vi "testPythonResults.vi"() -> ()   [LabVIEW 2011, in "run.lvlib"]
uses:
  run.lvlib
  Tools/Filing/FileReader/FileReader.lvclass
  Channels/Digital/DigitalOutput.lvclass
  Channels/DDSOutput/Generic/DDSOutput.lvclass
  Channels/VoltOutput/AnalogOutput.lvclass
panel:
  out "times":dbl[](array[numeric]) format="%#_6f"
  in  "Device":T1(ring)
  out "data":dbl[][](array[numeric])
  in  "Path":path=path "C:/Users/Administrator/Desktop/Crete/Data/2014/1411/141126/Scripts/Instrument Scripts/Dio64.csv"
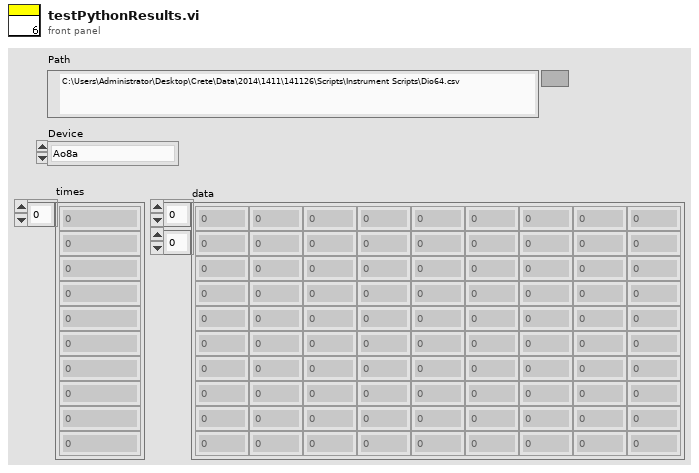
[diagram p1: front panel]
types:
  T1 = enum16{"Ao8a", "Ao8b", "Dio64", "K2602a", "K2602b", "K2602c", "K2602d", "SpinCoreDDS0", "SpinCoreDDS1"}
  T2 = cluster{"aoChannels":refnum<class "AnalogOutput.lvclass">[], "doChannels":refnum<class "DigitalOutput.lvclass">[], "rfChannels":refnum<class "DDSOutput.lvclass">[]}
  T3 = cluster{"Timestamps ms":dbl[], "DataPerChannel":dbl[][]}
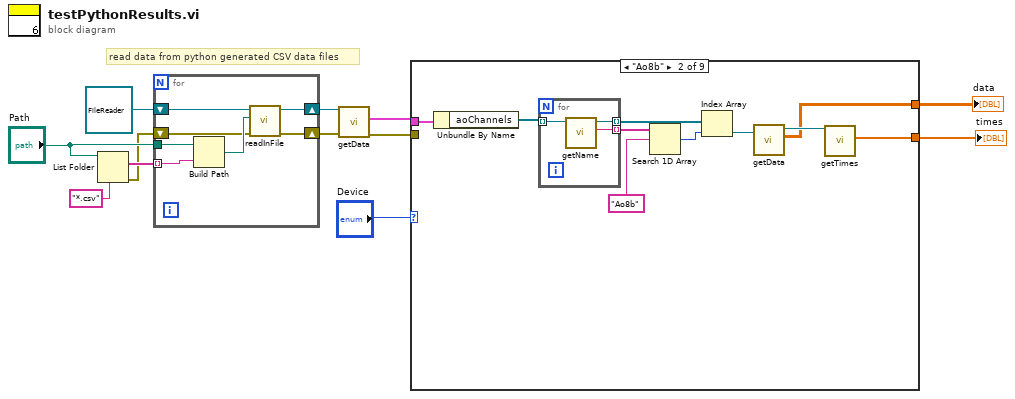
[diagram p0: block diagram]
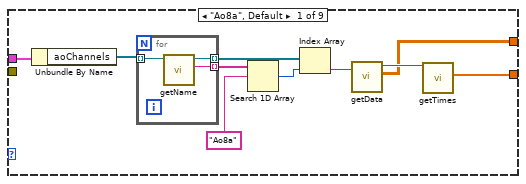
[diagram p2: hidden frame]
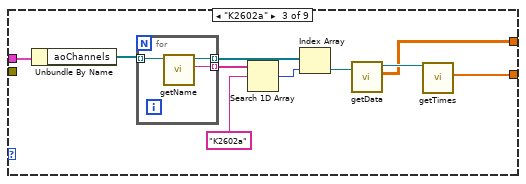
[diagram p3: hidden frame]
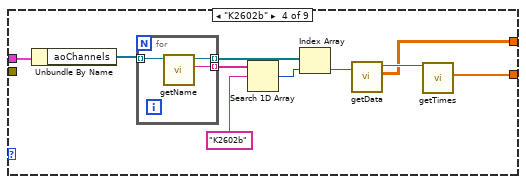
[diagram p4: hidden frame]
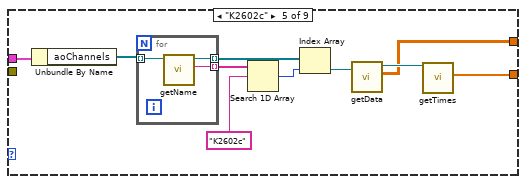
[diagram p5: hidden frame]
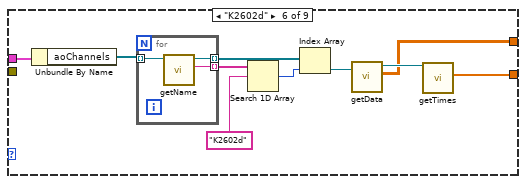
[diagram p6: hidden frame]
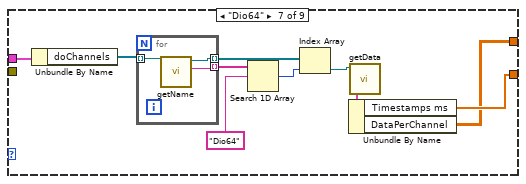
[diagram p7: hidden frame]
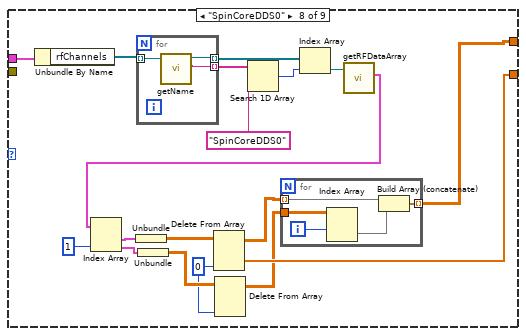
[diagram p8: hidden frame]
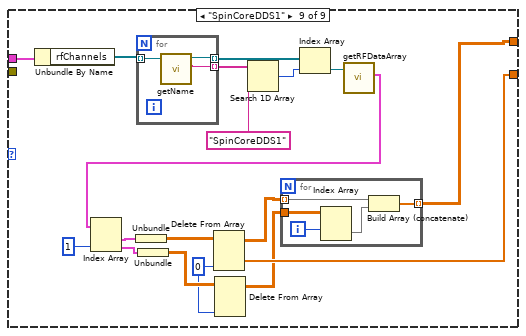
[diagram p9: hidden frame]
diagram:
  # "read data from python generated CSV data files"
  n1 = List Folder(path="Path", pattern="*.csv") -> (filenames=w11:string[], error out=w6:errorcluster)  [unwired: 2 in, 2 out]
  n2 = for {
    tunnel: "Path" -> [w18]
    tunnel: w11 -> [w19] mode=indexing
    shift-right: [w16] -> w9
    shift-left: refnum<class "FileReader.lvclass"> refnum ("FileReader out") -> [w14]
    shift-right: [w15] -> w8
    shift-left: w6 -> [w13]
    n3 = Build Path(base path=w18, name or relative path=w19) -> (appended path=w17:path)
    n4 = call "readInFile.vi"("error in (no error)"=w13, "Path"=w17, "FileReader in"=w14) -> ("error out"=w15:errorcluster, "FileReader out"=w16:refnum<class "FileReader.lvclass">)  [unwired: 7 in]
  }
  n5 = call "getData.vi"("error in (no error)"=w8, "FileReader in"=w9) -> ("error out"=w4:errorcluster, "Data"=w3:T2)  [unwired: 7 in, 1 out]
  n6 = case shown="\"Ao8b\"" "Device" {
    tunnel: w4 -> [_ _ _ _ _ _ _ _ _]
    tunnel: w3 -> [w29 w42 w55 w68 w81 w94 w107 w128 w154]
    tunnel: [w21 w34 w47 w60 w73 w86 w98 w111 w138] -> w2
    tunnel: [w20 w33 w46 w59 w72 w85 w99 w116 w143] -> w1
    frame "Ao8a", Default {
      n7 = Unbundle By Name(w29) -> ("aoChannels"=w28:refnum<class "AnalogOutput.lvclass">[])
      n8 = for {
        tunnel: w28 -> [w32] mode=indexing
        tunnel: [w31] -> w27 mode=indexing
        tunnel: [w30] -> w24 mode=indexing
        n9 = call "getName.vi"("AnalogOutput.lvclass in"=w32) -> ("name"=w31:string, "AnalogOutput.lvclass out"=w30:refnum<class "AnalogOutput.lvclass">)  [unwired: 8 in, 1 out]
      }
      n10 = Search 1D Array(1D array=w27, element="Ao8a") -> (index of element=w25:i32)  [unwired: 1 in]
      n11 = Index Array(array=w24, index=w25) -> (element=w23:refnum<class "AnalogOutput.lvclass">)
      n12 = call "getData.vi"("AnalogOutput.lvclass in"=w23) -> ("Data"=w21:dbl[][], "AnalogOutput.lvclass out"=w22:refnum<class "AnalogOutput.lvclass">)  [unwired: 8 in, 1 out]
      n13 = call "getTimes.vi"("AnalogOutput in"=w22) -> ("times"=w20:dbl[])  [unwired: 8 in, 2 out]
    }
    frame "Ao8b" {
      n14 = Unbundle By Name(w42) -> ("aoChannels"=w41:refnum<class "AnalogOutput.lvclass">[])
      n15 = for {
        tunnel: w41 -> [w45] mode=indexing
        tunnel: [w44] -> w40 mode=indexing
        tunnel: [w43] -> w37 mode=indexing
        n16 = call "getName.vi"("AnalogOutput.lvclass in"=w45) -> ("name"=w44:string, "AnalogOutput.lvclass out"=w43:refnum<class "AnalogOutput.lvclass">)  [unwired: 8 in, 1 out]
      }
      n17 = Search 1D Array(1D array=w40, element="Ao8b") -> (index of element=w38:i32)  [unwired: 1 in]
      n18 = Index Array(array=w37, index=w38) -> (element=w36:refnum<class "AnalogOutput.lvclass">)
      n19 = call "getData.vi"("AnalogOutput.lvclass in"=w36) -> ("Data"=w34:dbl[][], "AnalogOutput.lvclass out"=w35:refnum<class "AnalogOutput.lvclass">)  [unwired: 8 in, 1 out]
      n20 = call "getTimes.vi"("AnalogOutput in"=w35) -> ("times"=w33:dbl[])  [unwired: 8 in, 2 out]
    }
    frame "K2602a" {
      n21 = Unbundle By Name(w55) -> ("aoChannels"=w54:refnum<class "AnalogOutput.lvclass">[])
      n22 = for {
        tunnel: w54 -> [w58] mode=indexing
        tunnel: [w57] -> w53 mode=indexing
        tunnel: [w56] -> w50 mode=indexing
        n23 = call "getName.vi"("AnalogOutput.lvclass in"=w58) -> ("name"=w57:string, "AnalogOutput.lvclass out"=w56:refnum<class "AnalogOutput.lvclass">)  [unwired: 8 in, 1 out]
      }
      n24 = Search 1D Array(1D array=w53, element="K2602a") -> (index of element=w51:i32)  [unwired: 1 in]
      n25 = Index Array(array=w50, index=w51) -> (element=w49:refnum<class "AnalogOutput.lvclass">)
      n26 = call "getData.vi"("AnalogOutput.lvclass in"=w49) -> ("Data"=w47:dbl[][], "AnalogOutput.lvclass out"=w48:refnum<class "AnalogOutput.lvclass">)  [unwired: 8 in, 1 out]
      n27 = call "getTimes.vi"("AnalogOutput in"=w48) -> ("times"=w46:dbl[])  [unwired: 8 in, 2 out]
    }
    frame "K2602b" {
      n28 = Unbundle By Name(w68) -> ("aoChannels"=w67:refnum<class "AnalogOutput.lvclass">[])
      n29 = for {
        tunnel: w67 -> [w71] mode=indexing
        tunnel: [w70] -> w66 mode=indexing
        tunnel: [w69] -> w63 mode=indexing
        n30 = call "getName.vi"("AnalogOutput.lvclass in"=w71) -> ("name"=w70:string, "AnalogOutput.lvclass out"=w69:refnum<class "AnalogOutput.lvclass">)  [unwired: 8 in, 1 out]
      }
      n31 = Search 1D Array(1D array=w66, element="K2602b") -> (index of element=w64:i32)  [unwired: 1 in]
      n32 = Index Array(array=w63, index=w64) -> (element=w62:refnum<class "AnalogOutput.lvclass">)
      n33 = call "getData.vi"("AnalogOutput.lvclass in"=w62) -> ("Data"=w60:dbl[][], "AnalogOutput.lvclass out"=w61:refnum<class "AnalogOutput.lvclass">)  [unwired: 8 in, 1 out]
      n34 = call "getTimes.vi"("AnalogOutput in"=w61) -> ("times"=w59:dbl[])  [unwired: 8 in, 2 out]
    }
    frame "K2602c" {
      n35 = Unbundle By Name(w81) -> ("aoChannels"=w80:refnum<class "AnalogOutput.lvclass">[])
      n36 = for {
        tunnel: w80 -> [w84] mode=indexing
        tunnel: [w83] -> w79 mode=indexing
        tunnel: [w82] -> w76 mode=indexing
        n37 = call "getName.vi"("AnalogOutput.lvclass in"=w84) -> ("name"=w83:string, "AnalogOutput.lvclass out"=w82:refnum<class "AnalogOutput.lvclass">)  [unwired: 8 in, 1 out]
      }
      n38 = Search 1D Array(1D array=w79, element="K2602c") -> (index of element=w77:i32)  [unwired: 1 in]
      n39 = Index Array(array=w76, index=w77) -> (element=w75:refnum<class "AnalogOutput.lvclass">)
      n40 = call "getData.vi"("AnalogOutput.lvclass in"=w75) -> ("Data"=w73:dbl[][], "AnalogOutput.lvclass out"=w74:refnum<class "AnalogOutput.lvclass">)  [unwired: 8 in, 1 out]
      n41 = call "getTimes.vi"("AnalogOutput in"=w74) -> ("times"=w72:dbl[])  [unwired: 8 in, 2 out]
    }
    frame "K2602d" {
      n42 = Unbundle By Name(w94) -> ("aoChannels"=w93:refnum<class "AnalogOutput.lvclass">[])
      n43 = for {
        tunnel: w93 -> [w97] mode=indexing
        tunnel: [w96] -> w92 mode=indexing
        tunnel: [w95] -> w89 mode=indexing
        n44 = call "getName.vi"("AnalogOutput.lvclass in"=w97) -> ("name"=w96:string, "AnalogOutput.lvclass out"=w95:refnum<class "AnalogOutput.lvclass">)  [unwired: 8 in, 1 out]
      }
      n45 = Search 1D Array(1D array=w92, element="K2602d") -> (index of element=w90:i32)  [unwired: 1 in]
      n46 = Index Array(array=w89, index=w90) -> (element=w88:refnum<class "AnalogOutput.lvclass">)
      n47 = call "getData.vi"("AnalogOutput.lvclass in"=w88) -> ("Data"=w86:dbl[][], "AnalogOutput.lvclass out"=w87:refnum<class "AnalogOutput.lvclass">)  [unwired: 8 in, 1 out]
      n48 = call "getTimes.vi"("AnalogOutput in"=w87) -> ("times"=w85:dbl[])  [unwired: 8 in, 2 out]
    }
    frame "Dio64" {
      n49 = Unbundle By Name(w107) -> ("doChannels"=w106:refnum<class "DigitalOutput.lvclass">[])
      n50 = for {
        tunnel: w106 -> [w110] mode=indexing
        tunnel: [w108] -> w105 mode=indexing
        tunnel: [w109] -> w102 mode=indexing
        n51 = call-dynamic "getName.vi"("DigitalOutput.lvclass in"=w110) -> ("name"=w108:string, "DigitalOutput.lvclass out"=w109:refnum<class "DigitalOutput.lvclass">)  [unwired: 8 in, 1 out]
      }
      n52 = Search 1D Array(1D array=w105, element="Dio64") -> (index of element=w103:i32)  [unwired: 1 in]
      n53 = Index Array(array=w102, index=w103) -> (element=w101:refnum<class "DigitalOutput.lvclass">)
      n54 = call-dynamic "getData.vi"("DigitalOutput.lvclass in"=w101) -> ("Data"=w100:T3)  [unwired: 8 in, 2 out]
      n55 = Unbundle By Name(w100) -> ("Timestamps ms"=w99:dbl[], "DataPerChannel"=w98:dbl[][])
    }
    frame "SpinCoreDDS0" {
      w114 = 0 ("disabled index (col)")
      n56 = Unbundle By Name(w128) -> ("rfChannels"=w127:refnum<class "DDSOutput.lvclass">[])
      n57 = for {
        tunnel: w127 -> [w136] mode=indexing
        tunnel: [w134] -> w126 mode=indexing
        tunnel: [w135] -> w123 mode=indexing
        n58 = call-dynamic "getName.vi"("DDSOutput in"=w136) -> ("name"=w134:string, "DDSOutput out"=w135:refnum<class "DDSOutput.lvclass">)  [unwired: 8 in, 1 out]
      }
      n59 = Search 1D Array(1D array=w126, element="SpinCoreDDS0") -> (index of element=w124:i32)  [unwired: 1 in]
      n60 = Index Array(array=w123, index=w124) -> (element=w122:refnum<class "DDSOutput.lvclass">)
      n61 = call "getRFDataArray.vi"("DDSOutput in"=w122) -> ("rfDataArray"=w121:cluster{dbl[][]}[])  [unwired: 8 in, 2 out]
      n62 = Index Array(array=w121, index #2=1 ("index")) -> (element #1=w120:cluster{dbl[][]}, element #2=w119:cluster{dbl[][]})  [unwired: 1 in]
      n63 = Unbundle(w120) -> (w117:dbl[][])
      n64 = Unbundle(w119) -> (w115:dbl[][])
      n65 = Delete From Array(array=w117, index (col)=w114) -> (deleted portion=w116:dbl[], array with subset deleted=w113:dbl[][])  [unwired: 2 in]
      n66 = Delete From Array(array=w115, index (col)=w114) -> (array with subset deleted=w112:dbl[][])  [unwired: 2 in, 1 out]
      n67 = for {
        tunnel: w113 -> [w133] mode=indexing
        tunnel: w112 -> [w131]
        tunnel: [w132] -> w111 mode=indexing
        i -> [w130]
        n68 = Index Array(array=w131, index (row)=w130) -> (element=w129:dbl[])  [unwired: 1 in]
        n69 = Build Array (concatenate)(w133, w129) -> (w132:dbl[])
      }
    }
    frame "SpinCoreDDS1" {
      w141 = 0 ("disabled index (col)")
      n70 = Unbundle By Name(w154) -> ("rfChannels"=w153:refnum<class "DDSOutput.lvclass">[])
      n71 = for {
        tunnel: w153 -> [w162] mode=indexing
        tunnel: [w160] -> w152 mode=indexing
        tunnel: [w161] -> w149 mode=indexing
        n72 = call-dynamic "getName.vi"("DDSOutput in"=w162) -> ("name"=w160:string, "DDSOutput out"=w161:refnum<class "DDSOutput.lvclass">)  [unwired: 8 in, 1 out]
      }
      n73 = Search 1D Array(1D array=w152, element="SpinCoreDDS1") -> (index of element=w150:i32)  [unwired: 1 in]
      n74 = Index Array(array=w149, index=w150) -> (element=w148:refnum<class "DDSOutput.lvclass">)
      n75 = call "getRFDataArray.vi"("DDSOutput in"=w148) -> ("rfDataArray"=w137:cluster{dbl[][]}[])  [unwired: 8 in, 2 out]
      n76 = Index Array(array=w137, index #2=1 ("index")) -> (element #1=w147:cluster{dbl[][]}, element #2=w146:cluster{dbl[][]})  [unwired: 1 in]
      n77 = Unbundle(w147) -> (w144:dbl[][])
      n78 = Unbundle(w146) -> (w142:dbl[][])
      n79 = Delete From Array(array=w144, index (col)=w141) -> (deleted portion=w143:dbl[], array with subset deleted=w140:dbl[][])  [unwired: 2 in]
      n80 = Delete From Array(array=w142, index (col)=w141) -> (array with subset deleted=w139:dbl[][])  [unwired: 2 in, 1 out]
      n81 = for {
        tunnel: w140 -> [w157] mode=indexing
        tunnel: w139 -> [w158]
        tunnel: [w159] -> w138 mode=indexing
        i -> [w156]
        n82 = Index Array(array=w158, index (row)=w156) -> (element=w155:dbl[])  [unwired: 1 in]
        n83 = Build Array (concatenate)(w157, w155) -> (w159:dbl[])
      }
    }
  }
  "times" <- w1
  "data" <- w2
